vi "Test_PT1.vi"() -> ()   [LabVIEW 2022 SP3]
uses:
  AnalogSignalProcessClass.lvclass/AnalogSignalProcessClass.ctl
  <vilib>/measure/NI_MABase.lvlib
panel:
  out "XY Graph":cluster{dbl[], dbl[]}(graph)
  in  "sampling info":cluster{"Fs":dbl, "#s":dbl}={"Fs"=1000.0, "#s"=1000.0} {"Fs" format="%.2p"}
  in  "initialize":bool
  in  "T1":dbl
  in  "G":dbl
  in  "amplitude":dbl=1.0 format="%0.2p"
  in  "frequency":dbl=10.0 format="%0.2p"
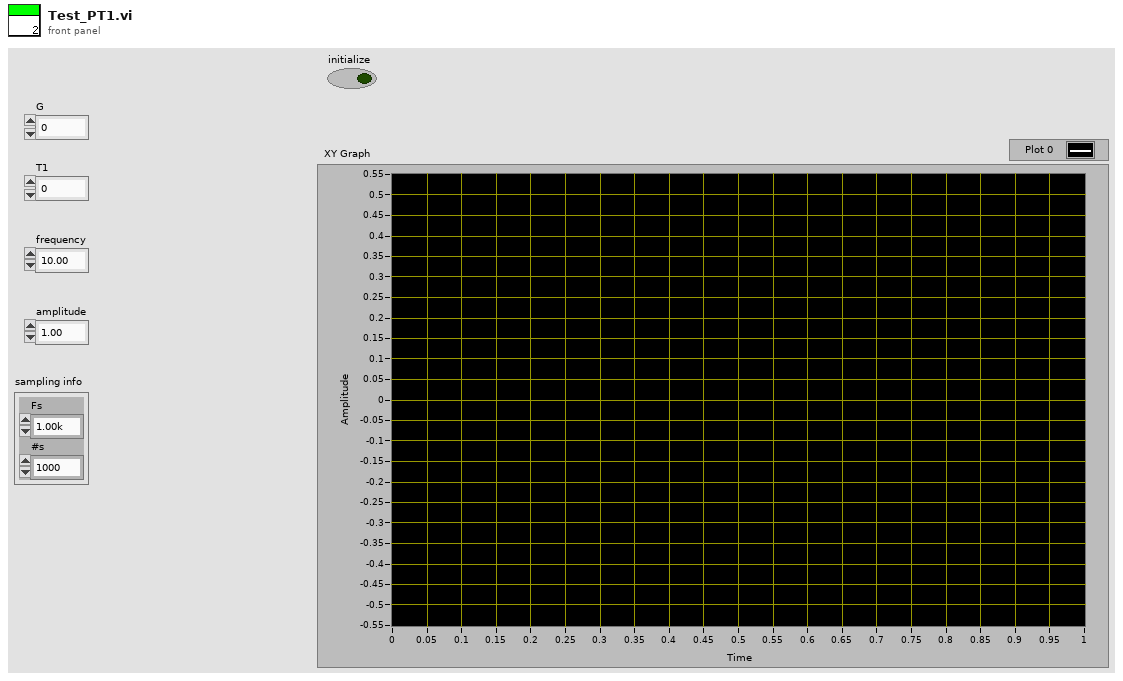
[diagram p1: front panel]
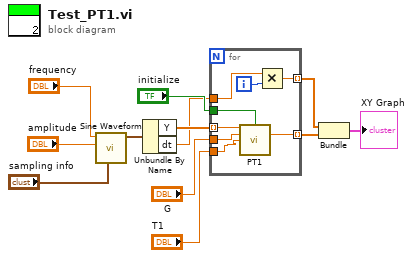
[diagram p0: block diagram]
diagram:
  n1 = call <vilib>:"Sine Waveform.vi"("sampling info"="sampling info", "amplitude"="amplitude", "frequency"="frequency") -> ("signal out"=w10:waveform(dbl))  [unwired: 7 in, 1 out]
  n2 = Unbundle By Name(w10) -> ("Y"=w9:dbl[], "dt"=w5:dbl)
  n3 = for {
    tunnel: w9 -> [w20] mode=indexing
    tunnel: "G" -> [w19]
    tunnel: "T1" -> [w13]
    tunnel: "initialize" -> [w18]
    tunnel: [w17] -> w2 mode=indexing
    tunnel: w5 -> [w15]
    tunnel: [w14] -> w3 mode=indexing
    i -> [w16]
    n4 = call "PT1.vi"("input u(k)"=w20, "initialize"=w18, "G"=w19, "T1"=w13) -> ("output y(k)"=w17:dbl)  [unwired: 10 in, 1 out]
    n5 = Multiply(x=w15, y=w16) -> (x*y=w14:dbl)
  }
  n6 = Bundle(w3, w2) -> (→"XY Graph":cluster{dbl[], dbl[]})  [unwired: 1 in]
